vi "Send GMail.vi"(8 "error in":errorcluster, 9 "Message":string, 10 "Subject":string="asdf", 11 "To:":string[](array[string])) -> (0 "error out":errorcluster)   [LabVIEW 2018]
doc: "Uses the SMTP Email Client to send an email to a standard or secure SMTP server."
uses:
  <vilib>/smtpClient/SmtpClientHandle.ctl
  <vilib>/smtpClient/Set Message Text.vi
  <vilib>/smtpClient/LabVIEWSMTPClient.lvlib
panel:
  out "Numeric":i32
  # "Compose Email"
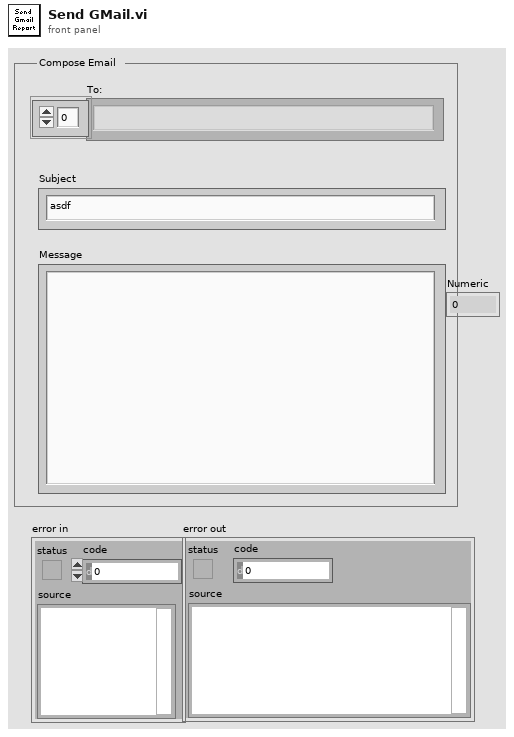
[diagram p1: front panel]
types:
  T1 = typedef "LabVIEWSMTPClient.lvlib/SmtpClientHandle.ctl" = refnum<k1>
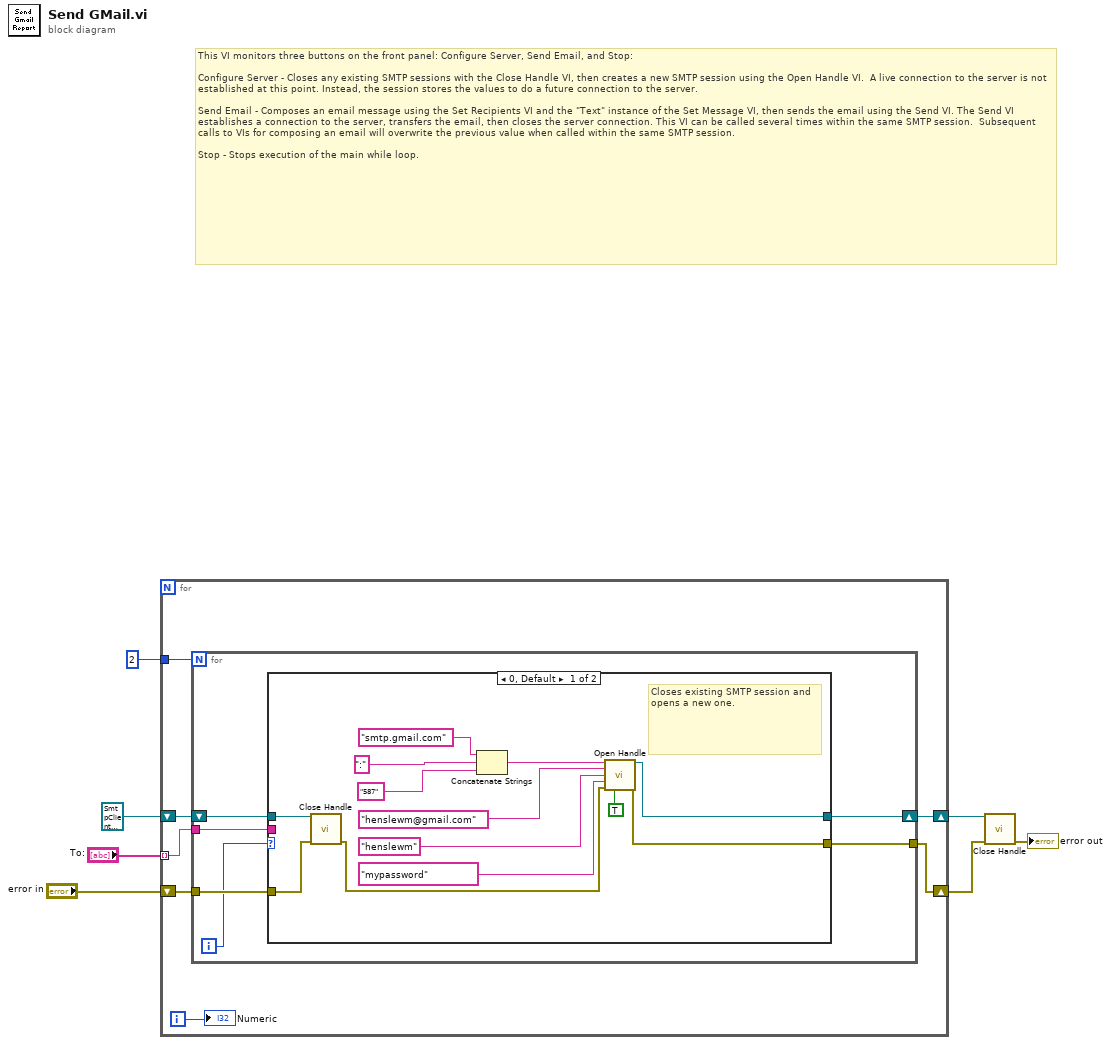
[diagram p0: block diagram]
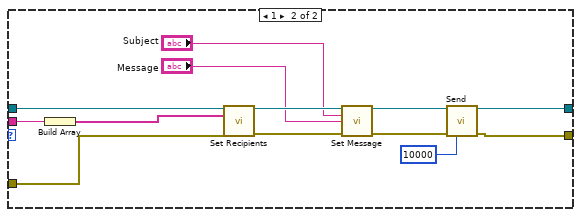
[diagram p2: hidden frame]
diagram:
  # "This VI monitors three buttons on the front panel: Configure Server, Send Email, and Stop:\n\nConfigure Server - Closes any existing SMTP sessions with the Close Handle VI, then creates a new SMTP session using the Open Handle VI.  A live connection to the server is not established at this point. Instead, the session stores the values to do a future connection to the server.\n\nSend Email - Composes an email message using the Set Recipients VI and the \"Text\" instance of the Set Message VI, then sends the email using the Send VI. The Send VI establishes a connection to the server, transfers the email, then closes the server connection. This VI can be called several times within the same SMTP session.  Subsequent calls to VIs for composing an email will overwrite the previous value when called within the same SMTP session.\n\nStop - Stops execution of the main while loop."
  n1 = for {
    tunnel: 2 -> [w10]
    shift-right: [w13] -> w5
    shift-left: T1 refnum ("handle out") -> [w14]
    shift-right: [w11] -> w3
    shift-left: "error in" -> [w12]
    tunnel: "To:" -> [w9] mode=indexing
    i -> [w8]
    n2 = for {
      N: w10 -> [_]
      shift-right: [w20] -> w13
      shift-left: w14 -> [w18]
      tunnel: w12 -> [w19]
      tunnel: [w17] -> w11
      tunnel: w9 -> [w15]
      i -> [w16]
      n3 = case shown="0, Default" w16 {
        tunnel: [w25 w36] -> w20
        tunnel: [w24 w37] -> w17
        tunnel: w19 -> [w22 w38]
        tunnel: w18 -> [w23 w39]
        tunnel: w15 -> [_ w35]
        frame 0, Default {
          # "Closes existing SMTP session and opens a new one."
          n4 = call <vilib>:"Close Handle.vi"("handle in"=w23, "error in (no error)"=w22) -> ("error out"=w21:errorcluster)  [unwired: 12 in, 1 out]
          n5 = Concatenate Strings("smtp.gmail.com" ("Outgoing Mail Server (SMTP)"), ":" ("string"), "587" ("Port")) -> (w30:string)
          n6 = call <vilib>:"Open Handle.vi"("server address"=w30, "from"="henslewm@gmail.com" ("Sender's Email Address"), "username"="henslewm" ("Username"), "password"="mypassword" ("Password"), "error in (no error)"=w21, "use TLS (false)"=TRUE ("Enable TLS")) -> ("handle out"=w25:T1, "error out"=w24:errorcluster)  [unwired: 8 in]
        }
        frame 1 {
          n7 = Build Array(w35) -> (w34:string[])
          n8 = call <vilib>:"Set Recipients.vi"("handle in"=w39, "to"=w34, "error in (no error)"=w38) -> ("handle out"=w43:T1, "error out"=w40:errorcluster)  [unwired: 11 in]
          n9 = call-poly <vilib>:"Set Message.vi"("handle in"=w43, "subject"="Subject", "plain text message"="Message", "error in (no error)"=w40) -> ("handle out"=w45:T1, "error out"=w44:errorcluster)  [unwired: 10 in]
          n10 = call <vilib>:"Send.vi"("handle in"=w45, "error in (no error)"=w44, "timeout in ms (10000)"=10000 ("timeout in ms")) -> ("handle out"=w36:T1, "error out"=w37:errorcluster)  [unwired: 10 in, 1 out]
        }
      }
    }
    "Numeric" <- w8
  }
  n11 = call <vilib>:"Close Handle.vi"("handle in"=w5, "error in (no error)"=w3) -> ("error out"=→"error out":errorcluster)  [unwired: 12 in, 1 out]
